vi "Convert_ERDs_Brass.vi"(0 "New Header?":bool, 7 "Array":T7[](array[typedef]) {"ERD Number" format="%.0x"}, 11 "Error In":errorcluster) -> (4 "All_ERD_Data_Bundled_Brass":T1, 15 "Error Out":errorcluster)   [LabVIEW 2016]
doc: "This VI parses the data from ERDs in correct format, units, etc. It handles all hex to dec conversions, hex to enum, and hex to boolean conversions.\n\nIf Raw Data from ERD is blank string, then it will output values from shift register."
uses:
  Common/LabVIEW GEA2 Toolkit/LabVIEW_GEA2_Toolkit.lvlibp/type defs/ERD Read Data Out.ctl
  type defs2/All_Bundled_Data_Brass.ctl
  Laundry Tool 1.0 Support/type defs/Version.ctl
  type defs2/ERD_Always_Show_Brass.ctl
  type defs2/CSV_File_String_Arrays.ctl
  type defs2/Fault Table Array.ctl
  Laundry Tool 1.0 Support/type defs/Fault_Table_Info.ctl
  Common/LabVIEW GEA2 Toolkit/LabVIEW_GEA2_Toolkit.lvlibp
panel:
  # "Software Version"
  # "UI"
  # "MC"
  # "INV"
  # "PERSONALITY"
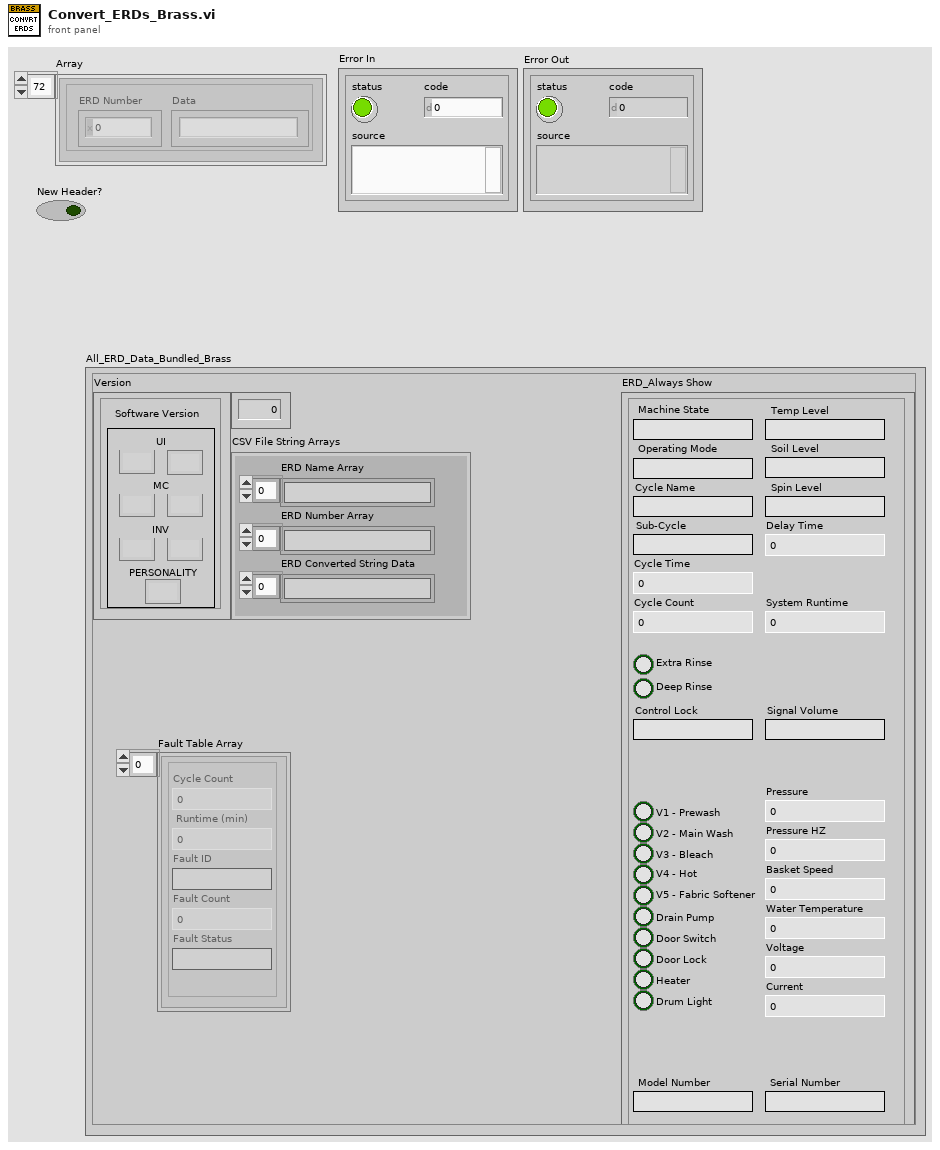
[diagram p1: front panel]
types:
  T1 = typedef "All_Bundled_Data_Brass.ctl" = cluster{"Version":T2, "ERD_Always Show":T3, "Personality Set":u8, "CSV File String Arrays":T4, "Fault Table Array ":T5}
  T2 = typedef "Version.ctl" = cluster{"UI Major":string, "UI Minor":string, "MC Minor":string, "MC Major":string, "Inverter Minor":string, "Inverter Major":string, "Personality":string}
  T3 = typedef "ERD_Always_Show_Brass.ctl" = cluster{"Machine State":string, "Cycle Count":u32, "Soil Level":string, "Spin Level":string, "Temp Level":string, "Delay Time":u16, "Sub-Cycle":string, "Cycle Name":string, "Model Number":string, "Serial Number":string, "System Runtime":u32, "Cycle Time":u16, "Operating Mode":string, "Deep Rinse":bool, "Extra Rinse":bool, "V1 - Prewash":bool, "V2 - Main Wash":bool, "V3 - Bleach":bool, "V4 - Hot":bool, "Drain Pump":bool, "Door Switch":bool, "Door Lock":bool, "Basket Speed":u16, "Water Temperature":dbl, "Voltage":u16, "Pressure":dbl, "Heater":bool, "Control Lock":string, "Signal Volume":string, "Current":u16, "Pressure HZ":dbl, "Drum Light":bool, "V5 - Fabric Softener":bool}
  T4 = typedef "CSV_File_String_Arrays.ctl" = cluster{"ERD Number Array":string[], "ERD Name Array":string[], "ERD Converted String Data":string[]}
  T5 = typedef "Fault Table Array.ctl" = T6[]
  T6 = typedef "Fault_Table_Info.ctl" = cluster{"Cycle Count":u32, " Runtime (min) ":u32, "Fault Status":string, "Fault ID":string, "Fault Count":u16}
  T7 = typedef "LabVIEW_GEA2_Toolkit.lvlibp/ERD Read Data Out.ctl" = cluster{"ERD Number":u16, "Data":string}
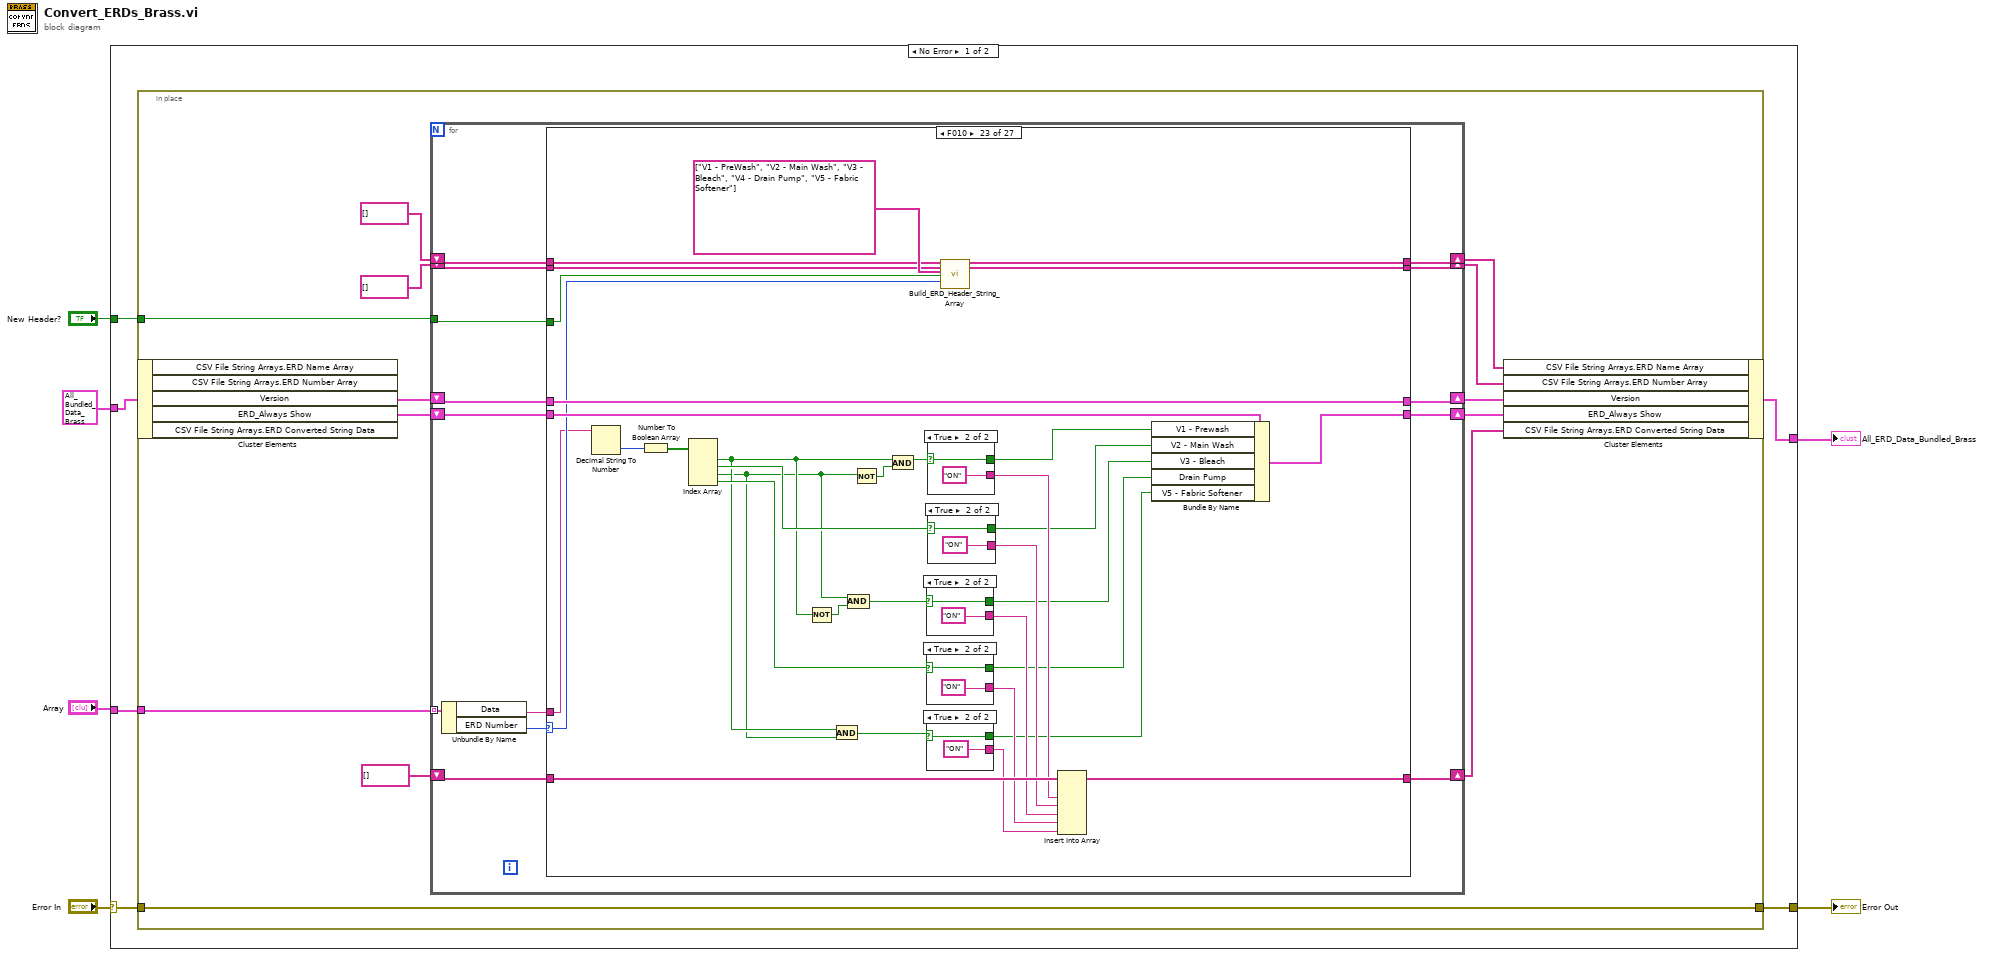
[diagram p0: block diagram]
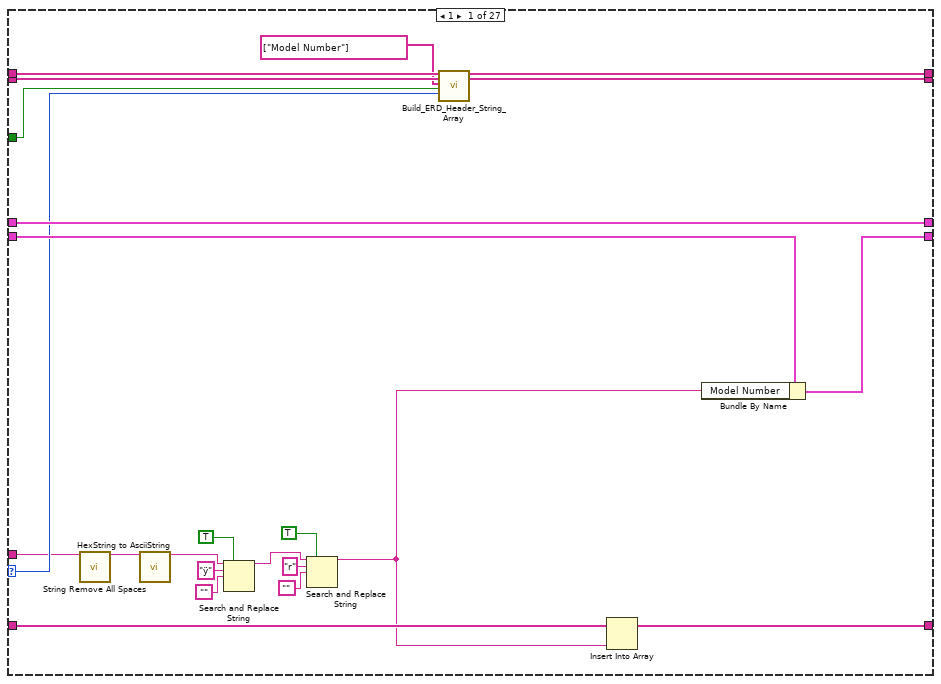
[diagram p2: hidden frame]
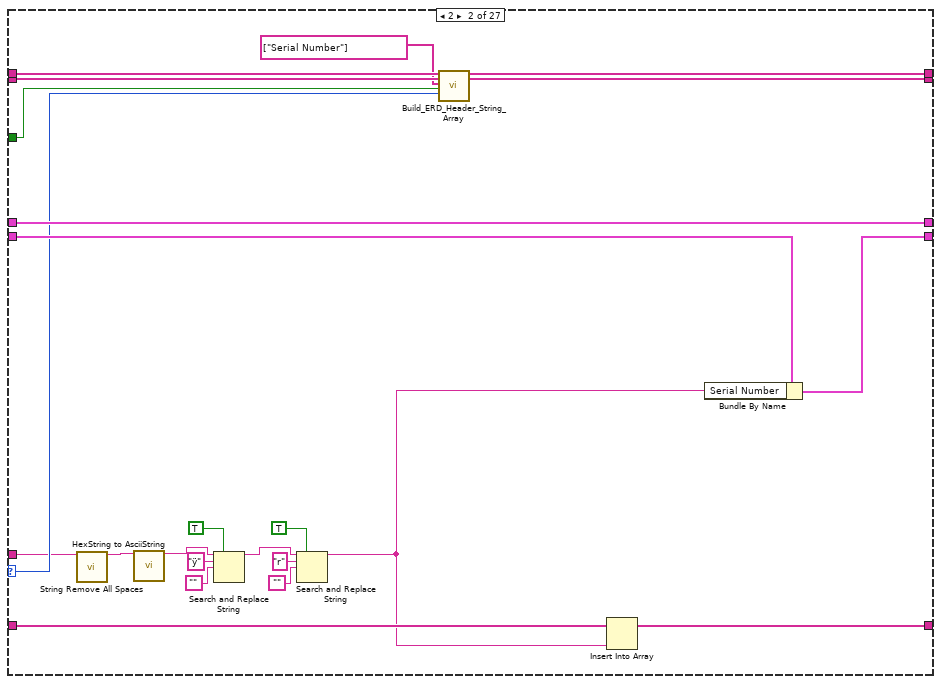
[diagram p3: hidden frame]
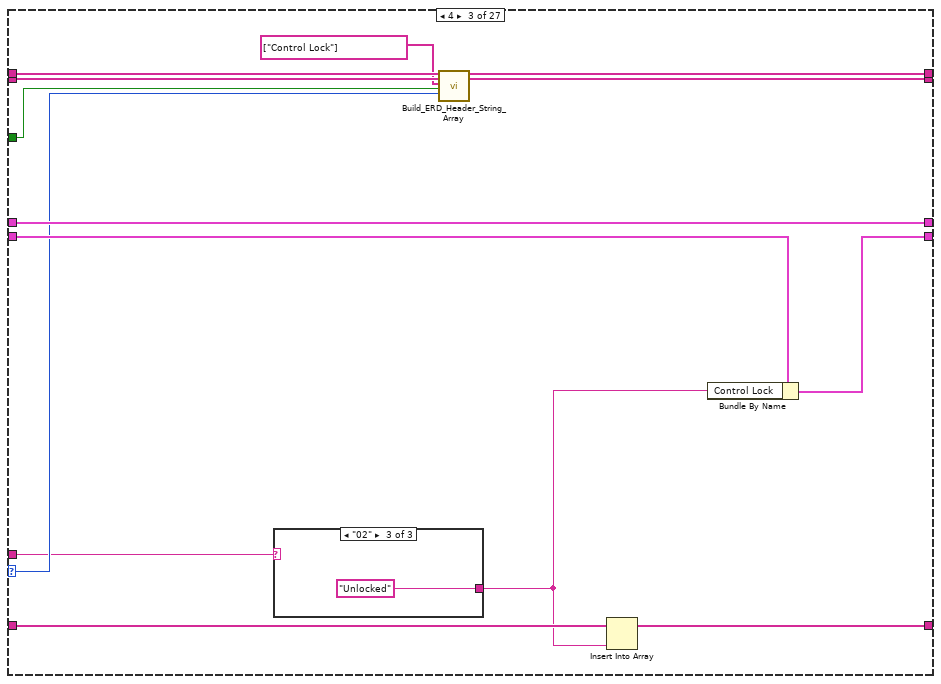
[diagram p4: hidden frame]
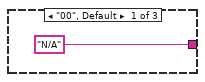
[diagram p5: hidden frame]
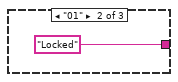
[diagram p6: hidden frame]
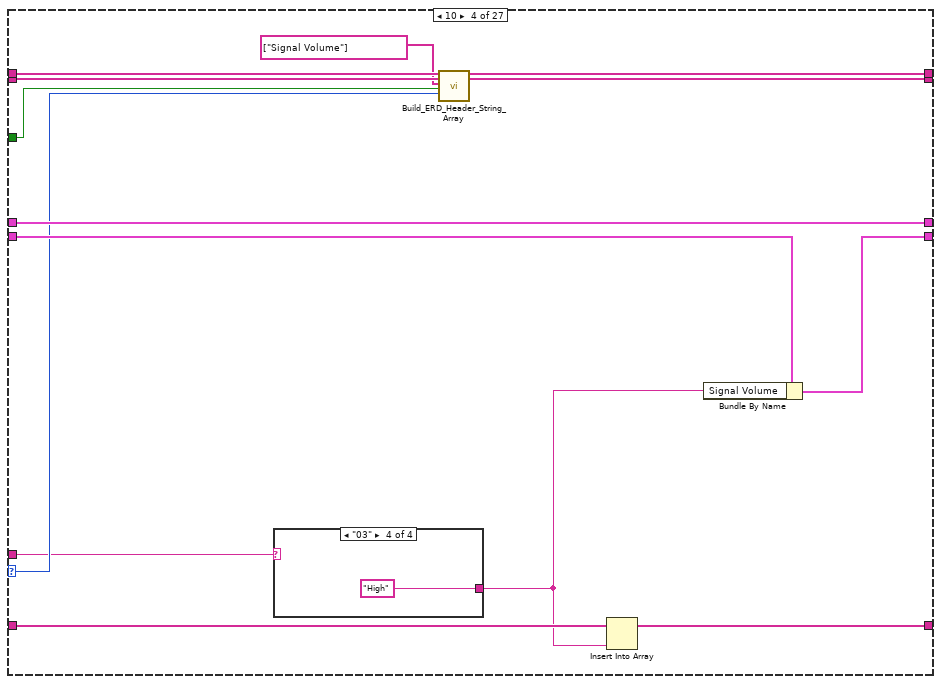
[diagram p7: hidden frame]
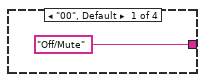
[diagram p8: hidden frame]
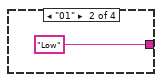
[diagram p9: hidden frame]
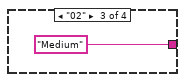
[diagram p10: hidden frame]
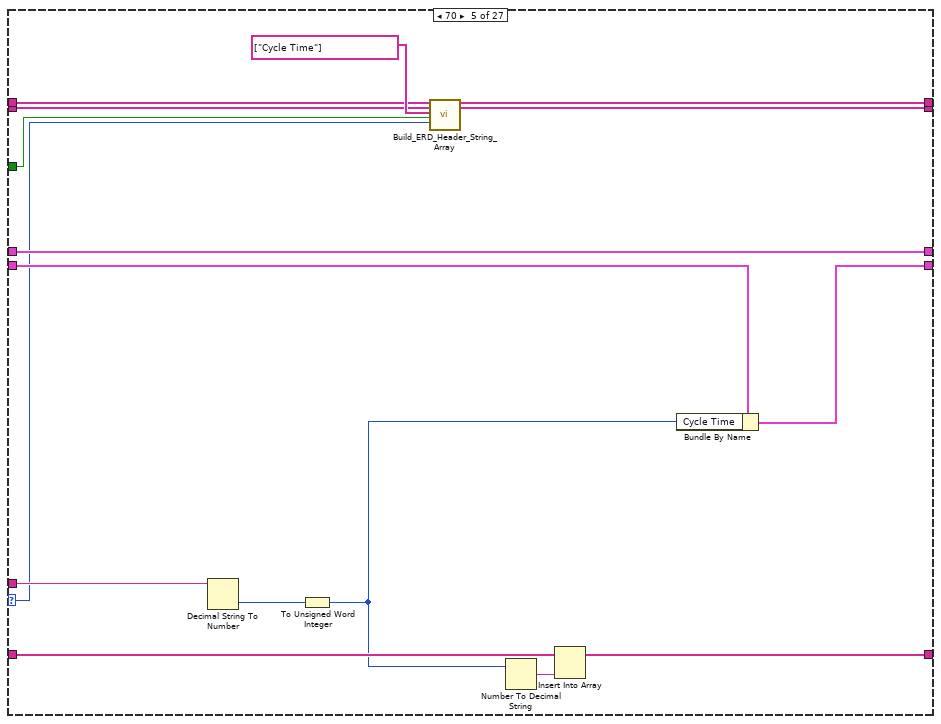
[diagram p11: hidden frame]
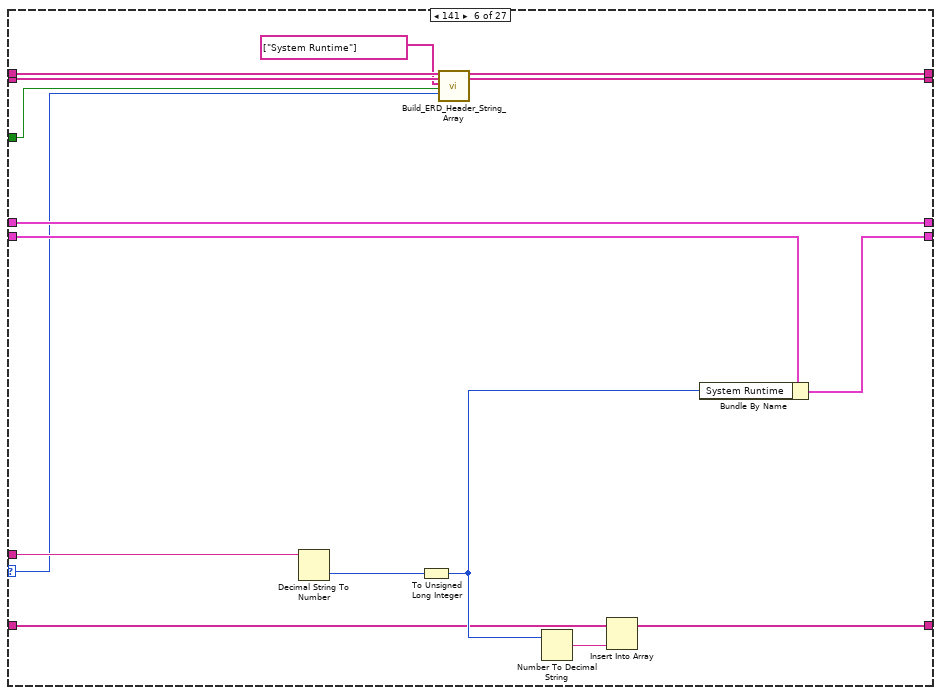
[diagram p12: hidden frame]
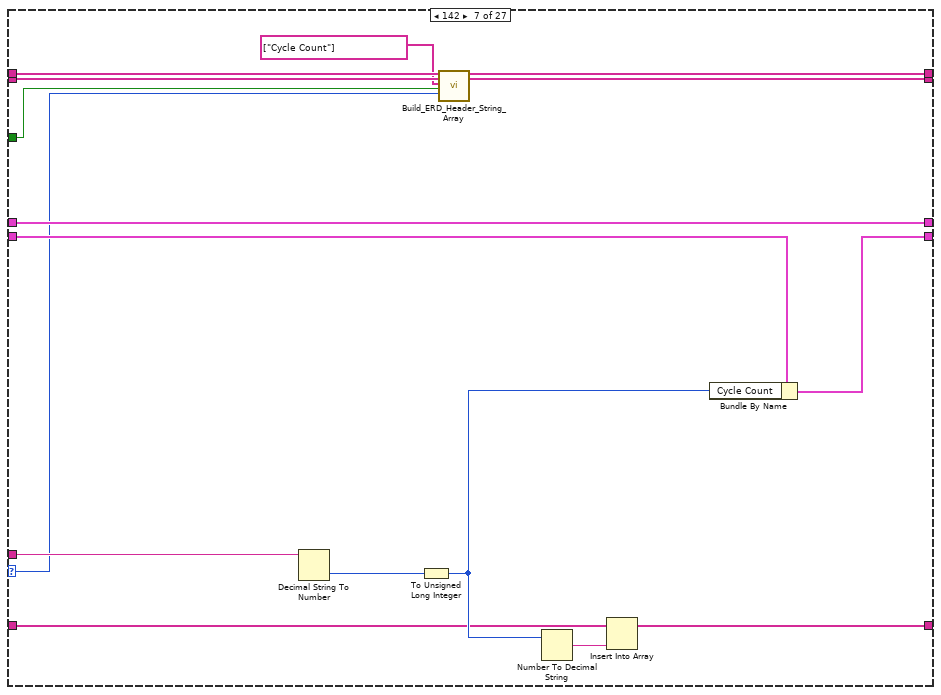
[diagram p13: hidden frame]
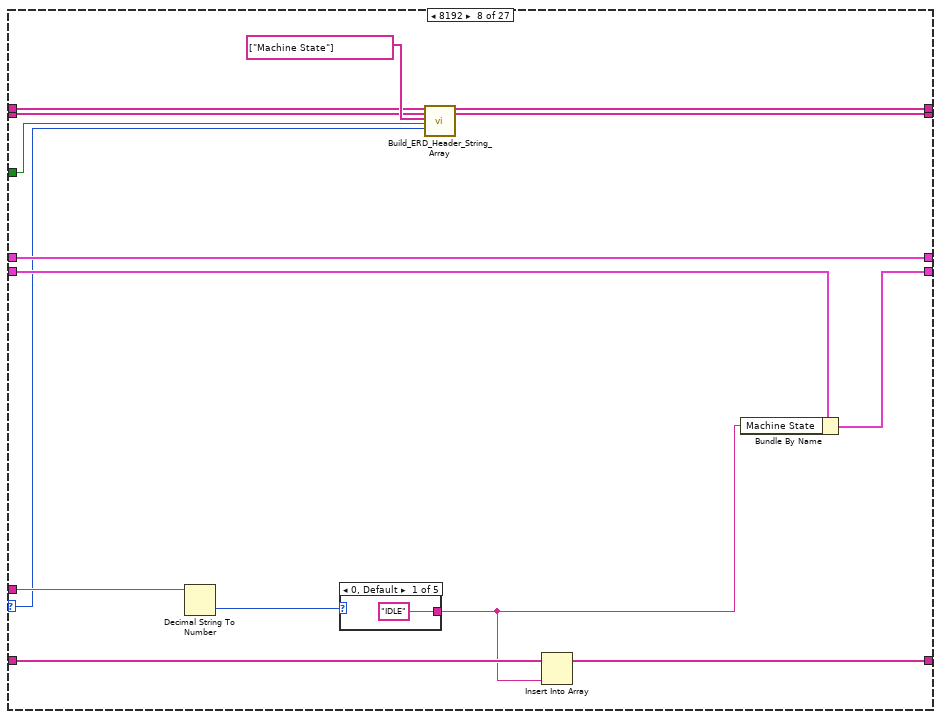
[diagram p14: hidden frame]
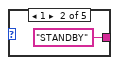
[diagram p15: hidden frame]
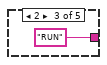
[diagram p16: hidden frame]
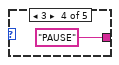
[diagram p17: hidden frame]
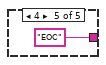
[diagram p18: hidden frame]
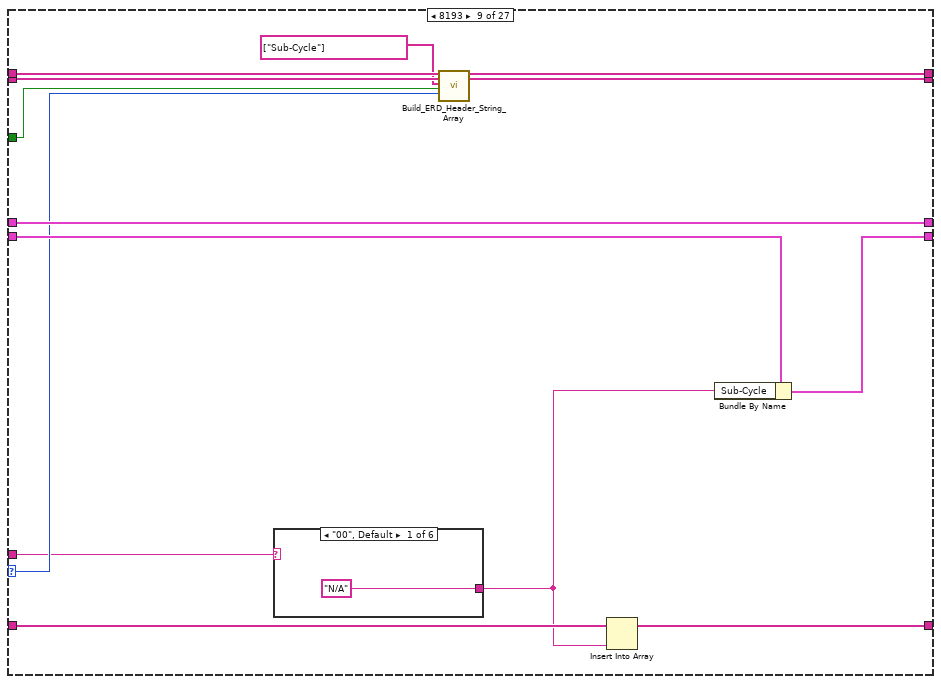
[diagram p19: hidden frame]
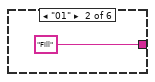
[diagram p20: hidden frame]
diagram:
  n1 = case shown="No Error" "Error In" {
    selector: "Error In" -> [w9 w657]
    tunnel: "Array" -> [w12 _]
    tunnel: [w10 w656] -> w4
    tunnel: T1 {"Version"={"UI Major"="", "UI Minor"="", "MC Minor"="", "MC Major"="", "Inverter Minor"="", "Inverter Major"="", "Personality"=""}, "ERD_Always Show"={"Machine State"="", "Cycle Count"=0, "Soil Level"="", "Spin Level"="", "Temp Level"="", "Delay Time"=0, "Sub-Cycle"="", "Cycle Name"="", "Model Number"="", "Serial Number"="", "System Runtime"=0, "Cycle Time"=0, "Operating Mode"="", "Deep Rinse"=FALSE, "Extra Rinse"=FALSE, "V1 - Prewash"=FALSE, "V2 - Main Wash"=FALSE, "V3 - Bleach"=FALSE, "V4 - Hot"=FALSE, "Drain Pump"=FALSE, "Door Switch"=FALSE, "Door Lock"=FALSE, "Basket Speed"=0, "Water Temperature"=0.0, "Voltage"=0, "Pressure"=0.0, "Heater"=FALSE, "Control Lock"="", "Signal Volume"="", "Current"=0, "Pressure HZ"=0.0, "Drum Light"=FALSE, "V5 - Fabric Softener"=FALSE}, "Personality Set"=0, "CSV File String Arrays"={"ERD Number Array"=[], "ERD Name Array"=[], "ERD Converted String Data"=[]}, "Fault Table Array "=[]} ("ERD_Data_Bundled_Out") -> [w11 w655]
    tunnel: [w8 w655] -> w3
    tunnel: "New Header?" -> [w7 _]
    frame No Error {
      n2 = in-place {
        in-place-border: w12 -> [w25]
        in-place-border: [w22] -> w10
        in-place-border: w9 -> [w22]
        in-place-border: w7 -> [w18]
        n3 = in-place-cluster #1(w11) -> ("Version"=w23:T2, "ERD_Always Show"=w24:T3)  [unwired: 3 out]
        n4 = for {
          tunnel: w25 -> [w39] mode=indexing
          shift-right: [w37] -> w20
          shift-left: w24 -> [w36]
          shift-right: [w34] -> w21
          shift-left: w23 -> [w35]
          shift-right: [w31] -> w13
          shift-left: string[] [] ("ERD String Data") -> [w32]
          tunnel: w18 -> [w30]
          shift-right: [w26] -> w14
          shift-left: string[] [] ("ERD String Data") -> [w29]
          shift-right: [w27] -> w15
          shift-left: string[] [] ("ERD String Data") -> [w28]
          n5 = Unbundle By Name(w39) -> ("Data"=w38:string, "ERD Number"=w33:u16)
          n6 = case shown="F010" w33 {
            selector: w33 -> [w53 w76 w90 w107 w121 w142 w158 w172 w193 w213 w270 w290 w311 w330 w344 w364 w387 w411 w442 w459 w478 w499 w537 w569 w588 w624 _]
            tunnel: w38 -> [w50 w73 w87 w104 w135 w152 w168 w180 w190 w210 w267 w304 w308 w327 w355 w375 w398 w421 w455 w472 w475 w498 w536 w583 w601 w603 _]
            tunnel: [w61 w84 w98 w115 w133 w150 w166 w183 w201 w221 w278 w302 w319 w338 w356 w376 w399 w422 w453 w470 w486 w509 w547 w581 w599 w635 w654] -> w37
            tunnel: w36 -> [w62 w85 w99 w116 w134 w151 w167 w182 w202 w222 w279 w303 w320 w339 w357 w377 w400 w423 w454 w471 w487 w510 w548 w582 w600 w635 w654]
            tunnel: w35 -> [w60 w83 w97 w114 w132 w149 w165 w179 w200 w220 w277 w301 w318 w337 w354 w374 w397 w420 w452 w469 w485 w508 w546 w580 w598 w637 w653]
            tunnel: [w60 w83 w97 w114 w132 w149 w165 w179 w200 w220 w277 w301 w318 w337 w354 w374 w397 w420 w452 w469 w485 w508 w546 w580 w598 w636 w653] -> w34
            tunnel: w32 -> [w58 w81 w95 w112 w125 w147 w163 w176 w198 w218 w275 w294 w316 w335 w348 w368 w391 w415 w446 w463 w483 w503 w541 w573 w592 w602 w651]
            tunnel: [w56 w79 w93 w110 w123 w145 w161 w174 w196 w216 w273 w292 w314 w333 w346 w366 w389 w413 w444 w461 w481 w501 w539 w571 w590 w626 w651] -> w31
            tunnel: w30 -> [w54 w77 w91 w108 w122 w143 w159 w173 w194 w214 w271 w291 w312 w331 w345 w365 w388 w412 w443 w460 w479 w500 w538 w570 w589 w625 _]
            tunnel: w29 -> [w59 w82 w96 w113 w126 w148 w164 w177 w199 w219 w276 w295 w317 w336 w349 w369 w392 w416 w447 w464 w484 w504 w542 w574 w593 w628 w652]
            tunnel: w28 -> [w52 w75 w89 w106 w130 w138 w154 w171 w192 w212 w269 w299 w310 w329 w353 w373 w396 w419 w450 w467 w477 w507 w545 w578 w596 w631 w650]
            tunnel: [w51 w74 w88 w105 w129 w137 w153 w170 w191 w211 w268 w298 w309 w328 w352 w372 w395 w418 w449 w466 w476 w506 w544 w577 w595 w630 w650] -> w27
            tunnel: [w57 w80 w94 w111 w124 w146 w162 w175 w197 w217 w274 w293 w315 w334 w347 w367 w390 w414 w445 w462 w482 w502 w540 w572 w591 w627 w652] -> w26
            frame 1 {
              n7 = call "String Remove All Spaces.vi"("Input String"=w50) -> ("Spaces Removed"=w49:string)  [unwired: 13 in, 1 out]
              n8 = call "HexString to AsciiString.vi"("Hex String"=w49) -> ("ASCII String"=w45:string)  [unwired: 13 in, 1 out]
              n9 = Search and Replace String(replace all?=TRUE ("replace all? (F)"), input string=w45, search string="ÿ", replace string="") -> (result string=w41:string)  [unwired: 4 in, 3 out]
              n10 = Search and Replace String(replace all?=TRUE ("replace all? (F)"), input string=w41, search string="r", replace string="") -> (result string=w44:string)  [unwired: 4 in, 3 out]
              n11 = call "Build_ERD_Header_String_Array.vi"("ERD Name Array In"=w59, "ERD Number Array In"=w58, "ERD Name List"=string[] ["Model Number"], "New Header?"=w54, "ERD Number"=w53) -> ("ERD Name Array Out"=w57:string[], "ERD Number Array Out"=w56:string[])  [unwired: 13 in]
              n12 = Insert Into Array(array=w52, new element=w44) -> (w51:string[])  [unwired: 1 in]
              n13 = Bundle By Name(cluster=w62, "Model Number"=w44) -> (w61:T3)
            }
            frame 2 {
              n14 = call "String Remove All Spaces.vi"("Input String"=w73) -> ("Spaces Removed"=w72:string)  [unwired: 13 in, 1 out]
              n15 = call "HexString to AsciiString.vi"("Hex String"=w72) -> ("ASCII String"=w69:string)  [unwired: 13 in, 1 out]
              n16 = Search and Replace String(replace all?=TRUE ("replace all? (F)"), input string=w69, search string="ÿ", replace string="") -> (result string=w64:string)  [unwired: 4 in, 3 out]
              n17 = Search and Replace String(replace all?=TRUE ("replace all? (F)"), input string=w64, search string="r", replace string="") -> (result string=w63:string)  [unwired: 4 in, 3 out]
              n18 = call "Build_ERD_Header_String_Array.vi"("ERD Name Array In"=w82, "ERD Number Array In"=w81, "ERD Name List"=string[] ["Serial Number"], "New Header?"=w77, "ERD Number"=w76) -> ("ERD Name Array Out"=w80:string[], "ERD Number Array Out"=w79:string[])  [unwired: 13 in]
              n19 = Insert Into Array(array=w75, new element=w63) -> (w74:string[])  [unwired: 1 in]
              n20 = Bundle By Name(cluster=w85, "Serial Number"=w63) -> (w84:T3)
            }
            frame 4 {
              n21 = case shown="\"02\"" w87 {
                tunnel: ["N/A" "Locked" "Unlocked"] -> w86
                frame "00", Default {
                }
                frame "01" {
                }
                frame "02" {
                }
              }
              n22 = call "Build_ERD_Header_String_Array.vi"("ERD Name Array In"=w96, "ERD Number Array In"=w95, "ERD Name List"=string[] ["Control Lock"], "New Header?"=w91, "ERD Number"=w90) -> ("ERD Name Array Out"=w94:string[], "ERD Number Array Out"=w93:string[])  [unwired: 13 in]
              n23 = Insert Into Array(array=w89, new element=w86) -> (w88:string[])  [unwired: 1 in]
              n24 = Bundle By Name(cluster=w99, "Control Lock"=w86) -> (w98:T3)
            }
            frame 10 {
              n25 = case shown="\"03\"" w104 {
                tunnel: ["Off/Mute" "Low" "Medium" "High"] -> w103
                frame "00", Default {
                }
                frame "01" {
                }
                frame "02" {
                }
                frame "03" {
                }
              }
              n26 = call "Build_ERD_Header_String_Array.vi"("ERD Name Array In"=w113, "ERD Number Array In"=w112, "ERD Name List"=string[] ["Signal Volume"], "New Header?"=w108, "ERD Number"=w107) -> ("ERD Name Array Out"=w111:string[], "ERD Number Array Out"=w110:string[])  [unwired: 13 in]
              n27 = Insert Into Array(array=w106, new element=w103) -> (w105:string[])  [unwired: 1 in]
              n28 = Bundle By Name(cluster=w116, "Signal Volume"=w103) -> (w115:T3)
            }
            frame 70 {
              n29 = Decimal String To Number(string=w135) -> (number=w136:i32)  [unwired: 2 in, 1 out]
              n30 = To Unsigned Word Integer(number=w136) -> (unsigned 16bit integer=w128:u16)
              n31 = call "Build_ERD_Header_String_Array.vi"("ERD Name Array In"=w126, "ERD Number Array In"=w125, "ERD Name List"=string[] ["Cycle Time"], "New Header?"=w122, "ERD Number"=w121) -> ("ERD Name Array Out"=w124:string[], "ERD Number Array Out"=w123:string[])  [unwired: 13 in]
              n32 = Number To Decimal String(number=w128) -> (decimal integer string=w131:string)  [unwired: 1 in]
              n33 = Insert Into Array(array=w130, new element=w131) -> (w129:string[])  [unwired: 1 in]
              n34 = Bundle By Name(cluster=w134, "Cycle Time"=w128) -> (w133:T3)
            }
            frame 141 {
              n35 = Decimal String To Number(string=w152) -> (number=w140:i32)  [unwired: 2 in, 1 out]
              n36 = To Unsigned Long Integer(number=w140) -> (unsigned 32bit integer=w139:u32)
              n37 = call "Build_ERD_Header_String_Array.vi"("ERD Name Array In"=w148, "ERD Number Array In"=w147, "ERD Name List"=string[] ["System Runtime"], "New Header?"=w143, "ERD Number"=w142) -> ("ERD Name Array Out"=w146:string[], "ERD Number Array Out"=w145:string[])  [unwired: 13 in]
              n38 = Number To Decimal String(number=w139) -> (decimal integer string=w141:string)  [unwired: 1 in]
              n39 = Insert Into Array(array=w138, new element=w141) -> (w137:string[])  [unwired: 1 in]
              n40 = Bundle By Name(cluster=w151, "System Runtime"=w139) -> (w150:T3)
            }
            frame 142 {
              n41 = Decimal String To Number(string=w168) -> (number=w156:i32)  [unwired: 2 in, 1 out]
              n42 = To Unsigned Long Integer(number=w156) -> (unsigned 32bit integer=w155:u32)
              n43 = call "Build_ERD_Header_String_Array.vi"("ERD Name Array In"=w164, "ERD Number Array In"=w163, "ERD Name List"=string[] ["Cycle Count"], "New Header?"=w159, "ERD Number"=w158) -> ("ERD Name Array Out"=w162:string[], "ERD Number Array Out"=w161:string[])  [unwired: 13 in]
              n44 = Number To Decimal String(number=w155) -> (decimal integer string=w157:string)  [unwired: 1 in]
              n45 = Insert Into Array(array=w154, new element=w157) -> (w153:string[])  [unwired: 1 in]
              n46 = Bundle By Name(cluster=w167, "Cycle Count"=w155) -> (w166:T3)
            }
            frame 8192 {
              n47 = Decimal String To Number(string=w180) -> (number=w181:i32)  [unwired: 2 in, 1 out]
              n48 = case shown="0, Default" w181 {
                tunnel: ["IDLE" "STANDBY" "RUN" "PAUSE" "EOC"] -> w169
                frame 0, Default {
                }
                frame 1 {
                }
                frame 2 {
                }
                frame 3 {
                }
                frame 4 {
                }
              }
              n49 = call "Build_ERD_Header_String_Array.vi"("ERD Name Array In"=w177, "ERD Number Array In"=w176, "ERD Name List"=string[] ["Machine State"], "New Header?"=w173, "ERD Number"=w172) -> ("ERD Name Array Out"=w175:string[], "ERD Number Array Out"=w174:string[])  [unwired: 13 in]
              n50 = Insert Into Array(array=w171, new element=w169) -> (w170:string[])  [unwired: 1 in]
              n51 = Bundle By Name(cluster=w182, "Machine State"=w169) -> (w183:T3)
            }
            frame 8193 {
              n52 = case shown="\"00\", Default" w190 {
                tunnel: ["N/A" "Fill" "Soak" "Wash" "Rinse" "Spin"] -> w189
                frame "00", Default {
                }
                frame "01" {
                }
                frame "02" {
                }
                frame "03" {
                }
                frame "04" {
                }
                frame "05" {
                }
              }
              n53 = call "Build_ERD_Header_String_Array.vi"("ERD Name Array In"=w199, "ERD Number Array In"=w198, "ERD Name List"=string[] ["Sub-Cycle"], "New Header?"=w194, "ERD Number"=w193) -> ("ERD Name Array Out"=w197:string[], "ERD Number Array Out"=w196:string[])  [unwired: 13 in]
              n54 = Insert Into Array(array=w192, new element=w189) -> (w191:string[])  [unwired: 1 in]
              n55 = Bundle By Name(cluster=w202, "Sub-Cycle"=w189) -> (w201:T3)
            }
            frame 8202 {
              n56 = case shown="\"19\"" w210 {
                tunnel: ["Not Defined" "Basket Clean" "Drain & Spin" "Quick Rinse" "Bulky Items" "Sanitize" "Towels & Sheets" "Steam Refresh" "Normal/Mixed" "Whites" "Dark Colors" "Jeans" "Hand Wash" "Delicates" "Speed Wash" "Heavy Duty" "Allergen" "Power Clean" "Rinse & Spin" "Single Item" "Colors" "Cold Wash" "Water on Demand" "Tub Clean" "Casuals w/ Steam" "Stain Wash w/ Steam" "Cottons" "Easy Care" "Active Wear" "Timed Dry" "Dewrinkle" "Air Fluff" "Steam Refresh" "Steam Dewrinkle" "Speed Dry" "Mixed" "Quick Dry" "Casuals" "Warm Up" "Energy Saver" "Antibacterial" "Rack Dry" "Baby Care"] -> w209
                frame "00", Default {
                }
                frame "01" {
                }
                frame "02" {
                }
                frame "03" {
                }
                frame "04" {
                }
                frame "05" {
                }
                frame "06" {
                }
                frame "07" {
                }
                frame "08" {
                }
                frame "09" {
                }
                frame "0A" {
                }
                frame "0B" {
                }
                frame "0C" {
                }
                frame "0D" {
                }
                frame "0E" {
                }
                frame "0F" {
                }
                frame "10" {
                }
                frame "11" {
                }
                frame "12" {
                }
                frame "13" {
                }
                frame "14" {
                }
                frame "15" {
                }
                frame "16" {
                }
                frame "17" {
                }
                frame "18" {
                }
                frame "19" {
                }
                frame "80" {
                }
                frame "81" {
                }
                frame "82" {
                }
                frame "83" {
                }
                frame "84" {
                }
                frame "85" {
                }
                frame "86" {
                }
                frame "87" {
                }
                frame "88" {
                }
                frame "89" {
                }
                frame "8A" {
                }
                frame "8B" {
                }
                frame "8C" {
                }
                frame "8D" {
                }
                frame "8E" {
                }
                frame "8F" {
                }
                frame "90" {
                }
              }
              n57 = call "Build_ERD_Header_String_Array.vi"("ERD Name Array In"=w219, "ERD Number Array In"=w218, "ERD Name List"=string[] ["Cycle Name"], "New Header?"=w214, "ERD Number"=w213) -> ("ERD Name Array Out"=w217:string[], "ERD Number Array Out"=w216:string[])  [unwired: 13 in]
              n58 = Insert Into Array(array=w212, new element=w209) -> (w211:string[])  [unwired: 1 in]
              n59 = Bundle By Name(cluster=w222, "Cycle Name"=w209) -> (w221:T3)
            }
            frame 8206 {
              n60 = case shown="\"09\"" w267 {
                tunnel: ["Consumer Mode" "Service Mode" "factory/EOL Mode" "Continuous Cycle Mode" "Rapid Relay Mode" "FCT Mode" "Model Plug" "Demo Mode" "Consumer Error Mode" "Floor Type Selection Mode"] -> w266
                frame "00", Default {
                }
                frame "01" {
                }
                frame "02" {
                }
                frame "03" {
                }
                frame "04" {
                }
                frame "05" {
                }
                frame "06" {
                }
                frame "07" {
                }
                frame "08" {
                }
                frame "09" {
                }
              }
              n61 = call "Build_ERD_Header_String_Array.vi"("ERD Name Array In"=w276, "ERD Number Array In"=w275, "ERD Name List"=string[] ["Operating Mode"], "New Header?"=w271, "ERD Number"=w270) -> ("ERD Name Array Out"=w274:string[], "ERD Number Array Out"=w273:string[])  [unwired: 13 in]
              n62 = Insert Into Array(array=w269, new element=w266) -> (w268:string[])  [unwired: 1 in]
              n63 = Bundle By Name(cluster=w279, "Operating Mode"=w266) -> (w278:T3)
            }
            frame 8208 {
              n64 = Decimal String To Number(string=w304) -> (number=w305:i32)  [unwired: 2 in, 1 out]
              n65 = To Unsigned Word Integer(number=w305) -> (unsigned 16bit integer=w297:u16)
              n66 = call "Build_ERD_Header_String_Array.vi"("ERD Name Array In"=w295, "ERD Number Array In"=w294, "ERD Name List"=string[] ["Delay Time"], "New Header?"=w291, "ERD Number"=w290) -> ("ERD Name Array Out"=w293:string[], "ERD Number Array Out"=w292:string[])  [unwired: 13 in]
              n67 = Number To Decimal String(number=w297) -> (decimal integer string=w300:string)  [unwired: 1 in]
              n68 = Insert Into Array(array=w299, new element=w300) -> (w298:string[])  [unwired: 1 in]
              n69 = Bundle By Name(cluster=w303, "Delay Time"=w297) -> (w302:T3)
            }
            frame 8210 {
              n70 = case shown="\"00\", Default" w308 {
                tunnel: ["Open" "Closed"] -> w307
                tunnel: [FALSE TRUE] -> w306
                frame "00", Default {
                }
                frame "01" {
                }
              }
              n71 = call "Build_ERD_Header_String_Array.vi"("ERD Name Array In"=w317, "ERD Number Array In"=w316, "ERD Name List"=string[] ["Door Switch"], "New Header?"=w312, "ERD Number"=w311) -> ("ERD Name Array Out"=w315:string[], "ERD Number Array Out"=w314:string[])  [unwired: 13 in]
              n72 = Insert Into Array(array=w310, new element=w307) -> (w309:string[])  [unwired: 1 in]
              n73 = Bundle By Name(cluster=w320, "Door Switch"=w306) -> (w319:T3)
            }
            frame 8211 {
              n74 = case shown="\"01\"" w327 {
                tunnel: ["Unlocked" "Locked"] -> w326
                tunnel: [FALSE TRUE] -> w325
                frame "00", Default {
                }
                frame "01" {
                }
              }
              n75 = call "Build_ERD_Header_String_Array.vi"("ERD Name Array In"=w336, "ERD Number Array In"=w335, "ERD Name List"=string[] ["Door Lock"], "New Header?"=w331, "ERD Number"=w330) -> ("ERD Name Array Out"=w334:string[], "ERD Number Array Out"=w333:string[])  [unwired: 13 in]
              n76 = Insert Into Array(array=w329, new element=w326) -> (w328:string[])  [unwired: 1 in]
              n77 = Bundle By Name(cluster=w339, "Door Lock"=w325) -> (w338:T3)
            }
            frame 8213 {
              n78 = case shown="\"00\"" w355 {
                selector: w355 -> [w358 _ _ _ _ _]
                tunnel: [w358 "Extra Light" "Light" "Normal" "Heavy" "Extra Heavy"] -> w351
                frame Default {
                }
                frame "00" {
                }
                frame "01" {
                }
                frame "02" {
                }
                frame "03" {
                }
                frame "04" {
                }
              }
              n79 = call "Build_ERD_Header_String_Array.vi"("ERD Name Array In"=w349, "ERD Number Array In"=w348, "ERD Name List"=string[] ["Soil Level"], "New Header?"=w345, "ERD Number"=w344) -> ("ERD Name Array Out"=w347:string[], "ERD Number Array Out"=w346:string[])  [unwired: 13 in]
              n80 = Insert Into Array(array=w353, new element=w351) -> (w352:string[])  [unwired: 1 in]
              n81 = Bundle By Name(cluster=w357, "Soil Level"=w351) -> (w356:T3)
            }
            frame 8214 {
              n82 = case shown="\"22\"" w375 {
                selector: w375 -> [w378 _ _ _ _ _ _ _ _]
                tunnel: [w378 "Disabled" "Tap Cold" "Cold" "Cool" "Colors" "Warm" "Hot" "Extra Hot"] -> w371
                frame Default {
                }
                frame "06" {
                }
                frame "16" {
                }
                frame "17" {
                }
                frame "18" {
                }
                frame "19" {
                }
                frame "20" {
                }
                frame "21" {
                }
                frame "22" {
                }
              }
              n83 = call "Build_ERD_Header_String_Array.vi"("ERD Name Array In"=w369, "ERD Number Array In"=w368, "ERD Name List"=string[] ["Temp Level"], "New Header?"=w365, "ERD Number"=w364) -> ("ERD Name Array Out"=w367:string[], "ERD Number Array Out"=w366:string[])  [unwired: 13 in]
              n84 = Insert Into Array(array=w373, new element=w371) -> (w372:string[])  [unwired: 1 in]
              n85 = Bundle By Name(cluster=w377, "Temp Level"=w371) -> (w376:T3)
            }
            frame 8215 {
              n86 = case shown="\"5\"" w398 {
                selector: w398 -> [w401 _ _ _ _ _ _]
                tunnel: [w401 "No Spin" "Low" "Medium" "High" "Extra High" "Disable"] -> w394
                frame Default {
                }
                frame "0" {
                }
                frame "1" {
                }
                frame "2" {
                }
                frame "3" {
                }
                frame "4" {
                }
                frame "5" {
                }
              }
              n87 = call "Build_ERD_Header_String_Array.vi"("ERD Name Array In"=w392, "ERD Number Array In"=w391, "ERD Name List"=string[] ["Spin Level"], "New Header?"=w388, "ERD Number"=w387) -> ("ERD Name Array Out"=w390:string[], "ERD Number Array Out"=w389:string[])  [unwired: 13 in]
              n88 = Insert Into Array(array=w396, new element=w394) -> (w395:string[])  [unwired: 1 in]
              n89 = Bundle By Name(cluster=w400, "Spin Level"=w394) -> (w399:T3)
            }
            frame 8216 {
              n90 = case shown="\"3\"" w421 {
                selector: w421 -> [w424 _ _ _ _]
                tunnel: [w424 "0 - Deep Rinse OFF - Extra Rinse OFF" "1 - Deep Rinse ON - Extra Rinse OFF" "2 - Deep Rinse OFF - Extra Rinse ON" "3 - Deep Rinse ON - Extra Rinse ON"] -> w410
                tunnel: [FALSE FALSE TRUE FALSE TRUE] -> w409
                tunnel: [FALSE FALSE FALSE TRUE TRUE] -> w408
                frame Default {
                }
                frame "0" {
                }
                frame "1" {
                }
                frame "2" {
                }
                frame "3" {
                }
              }
              n91 = call "Build_ERD_Header_String_Array.vi"("ERD Name Array In"=w416, "ERD Number Array In"=w415, "ERD Name List"=string[] ["Rinse Options"], "New Header?"=w412, "ERD Number"=w411) -> ("ERD Name Array Out"=w414:string[], "ERD Number Array Out"=w413:string[])  [unwired: 13 in]
              n92 = Insert Into Array(array=w419, new element=w410) -> (w418:string[])  [unwired: 1 in]
              n93 = Bundle By Name(cluster=w423, "Deep Rinse"=w409, "Extra Rinse"=w408) -> (w422:T3)
            }
            frame 8258 {
              n94 = Decimal String To Number(string=w455) -> (number=w441:i32)  [unwired: 2 in, 1 out]
              n95 = Divide(x=w441, y=1000) -> (x/y=w439:dbl)
              n96 = call "Build_ERD_Header_String_Array.vi"("ERD Name Array In"=w447, "ERD Number Array In"=w446, "ERD Name List"=string[] ["Pressure"], "New Header?"=w443, "ERD Number"=w442) -> ("ERD Name Array Out"=w445:string[], "ERD Number Array Out"=w444:string[])  [unwired: 13 in]
              n97 = Number To Fractional String(number=w439) -> (F-format string=w451:string)  [unwired: 3 in]
              n98 = Insert Into Array(array=w450, new element=w451) -> (w449:string[])  [unwired: 1 in]
              n99 = Bundle By Name(cluster=w454, "Pressure"=w439) -> (w453:T3)
            }
            frame 8259 {
              n100 = Decimal String To Number(string=w472) -> (number=w458:i32)  [unwired: 2 in, 1 out]
              n101 = Divide(x=w458, y=10) -> (x/y=w456:dbl)
              n102 = call "Build_ERD_Header_String_Array.vi"("ERD Name Array In"=w464, "ERD Number Array In"=w463, "ERD Name List"=string[] ["Water Temperature"], "New Header?"=w460, "ERD Number"=w459) -> ("ERD Name Array Out"=w462:string[], "ERD Number Array Out"=w461:string[])  [unwired: 13 in]
              n103 = Number To Fractional String(number=w456) -> (F-format string=w468:string)  [unwired: 3 in]
              n104 = Insert Into Array(array=w467, new element=w468) -> (w466:string[])  [unwired: 1 in]
              n105 = Bundle By Name(cluster=w471, "Water Temperature"=w456) -> (w470:T3)
            }
            frame 61452 {
              n106 = case shown="\"01\"" w475 {
                tunnel: ["OFF" "ON"] -> w474
                tunnel: [FALSE TRUE] -> w473
                frame "00", Default {
                }
                frame "01" {
                }
              }
              n107 = call "Build_ERD_Header_String_Array.vi"("ERD Name Array In"=w484, "ERD Number Array In"=w483, "ERD Name List"=string[] ["Drum Light"], "New Header?"=w479, "ERD Number"=w478) -> ("ERD Name Array Out"=w482:string[], "ERD Number Array Out"=w481:string[])  [unwired: 13 in]
              n108 = Insert Into Array(array=w477, new element=w474) -> (w476:string[])  [unwired: 1 in]
              n109 = Bundle By Name(cluster=w487, "Drum Light"=w473) -> (w486:T3)
            }
            frame 61455 {
              n110 = Decimal String To Number(string=w498) -> (number=w497:i32)  [unwired: 2 in, 1 out]
              n111 = Number To Boolean Array(number=w497) -> (Boolean array=w496:bool[])
              n112 = Index Array(array=w496) -> (element #2=w493:bool, element #6=w492:bool)  [unwired: 6 in, 4 out]
              n113 = case shown="True" w493 {
                tunnel: ["OFF" "ON"] -> w495
                frame False {
                }
                frame True {
                }
              }
              n114 = case shown="True" w492 {
                tunnel: ["OFF" "ON"] -> w494
                frame False {
                }
                frame True {
                }
              }
              n115 = call "Build_ERD_Header_String_Array.vi"("ERD Name Array In"=w504, "ERD Number Array In"=w503, "ERD Name List"=string[] ["Heater", "V4 - Hot"], "New Header?"=w500, "ERD Number"=w499) -> ("ERD Name Array Out"=w502:string[], "ERD Number Array Out"=w501:string[])  [unwired: 13 in]
              n116 = Insert Into Array(array=w507, new element #1=w495, new element #2=w494) -> (w506:string[])  [unwired: 1 in]
              n117 = Bundle By Name(cluster=w510, "Heater"=w493, "V4 - Hot"=w492) -> (w509:T3)
            }
            frame 61456 {
              n118 = Decimal String To Number(string=w536) -> (number=w535:i32)  [unwired: 2 in, 1 out]
              n119 = Number To Boolean Array(number=w535) -> (Boolean array=w534:bool[])
              n120 = Index Array(array=w534) -> (element #1=w520:bool, element #2=w529:bool, element #3=w519:bool, element #4=w525:bool)  [unwired: 4 in]
              n121 = Not(x=w520) -> (.not. x?=w524:bool)
              n122 = And(x=w520, y=w519) -> (x .and. y?=w521:bool)
              n123 = And(x=w519, y=w524) -> (x .and. y?=w523:bool)
              n124 = Not(x=w519) -> (.not. x?=w527:bool)
              n125 = And(x=w520, y=w527) -> (x .and. y?=w528:bool)
              n126 = case shown="True" w523 {
                selector: w523 -> [w557 w559]
                tunnel: ["OFF" "ON"] -> w531
                tunnel: [w557 w559] -> w522
                frame False {
                }
                frame True {
                }
              }
              n127 = case shown="True" w525 {
                selector: w525 -> [w553 w555]
                tunnel: ["OFF" "ON"] -> w530
                tunnel: [w553 w555] -> w517
                frame False {
                }
                frame True {
                }
              }
              n128 = case shown="True" w521 {
                selector: w521 -> [w549 w551]
                tunnel: ["OFF" "ON"] -> w515
                tunnel: [w549 w551] -> w518
                frame False {
                }
                frame True {
                }
              }
              n129 = case shown="True" w528 {
                selector: w528 -> [w565 w567]
                tunnel: ["OFF" "ON"] -> w533
                tunnel: [w565 w567] -> w526
                frame False {
                }
                frame True {
                }
              }
              n130 = case shown="True" w529 {
                selector: w529 -> [w561 w563]
                tunnel: ["OFF" "ON"] -> w532
                tunnel: [w561 w563] -> w516
                frame False {
                }
                frame True {
                }
              }
              n131 = call "Build_ERD_Header_String_Array.vi"("ERD Name Array In"=w542, "ERD Number Array In"=w541, "ERD Name List"=string[] ["V1 - PreWash", "V2 - Main Wash", "V3 - Bleach", "V4 - Drain Pump", "V5 - Fabric Softener"], "New Header?"=w538, "ERD Number"=w537) -> ("ERD Name Array Out"=w540:string[], "ERD Number Array Out"=w539:string[])  [unwired: 13 in]
              n132 = Insert Into Array(array=w545, new element #1=w533, new element #2=w532, new element #3=w531, new element #4=w530, new element #5=w515) -> (w544:string[])  [unwired: 1 in]
              n133 = Bundle By Name(cluster=w548, "V1 - Prewash"=w526, "V2 - Main Wash"=w516, "V3 - Bleach"=w522, "Drain Pump"=w517, "V5 - Fabric Softener"=w518) -> (w547:T3)
            }
            frame 61457 {
              n134 = Decimal String To Number(string=w583) -> (number=w584:i32)  [unwired: 2 in, 1 out]
              n135 = To Unsigned Word Integer(number=w584) -> (unsigned 16bit integer=w576:u16)
              n136 = call "Build_ERD_Header_String_Array.vi"("ERD Name Array In"=w574, "ERD Number Array In"=w573, "ERD Name List"=string[] ["Basket Speed"], "New Header?"=w570, "ERD Number"=w569) -> ("ERD Name Array Out"=w572:string[], "ERD Number Array Out"=w571:string[])  [unwired: 13 in]
              n137 = Number To Decimal String(number=w576) -> (decimal integer string=w579:string)  [unwired: 1 in]
              n138 = Insert Into Array(array=w578, new element=w579) -> (w577:string[])  [unwired: 1 in]
              n139 = Bundle By Name(cluster=w582, "Basket Speed"=w576) -> (w581:T3)
            }
            frame 61458 {
              n140 = Decimal String To Number(string=w601) -> (number=w587:i32)  [unwired: 2 in, 1 out]
              n141 = Divide(x=w587, y=100) -> (x/y=w585:dbl)
              n142 = call "Build_ERD_Header_String_Array.vi"("ERD Name Array In"=w593, "ERD Number Array In"=w592, "ERD Name List"=string[] ["Pressure Hz"], "New Header?"=w589, "ERD Number"=w588) -> ("ERD Name Array Out"=w591:string[], "ERD Number Array Out"=w590:string[])  [unwired: 13 in]
              n143 = Number To Fractional String(number=w585) -> (F-format string=w597:string)  [unwired: 3 in]
              n144 = Insert Into Array(array=w596, new element=w597) -> (w595:string[])  [unwired: 1 in]
              n145 = Bundle By Name(cluster=w600, "Pressure HZ"=w585) -> (w599:T3)
            }
            frame 61460 {
              w613 = 2 ("length (rest)")
              n146 = String Subset(string=w603, offset (0)=0 ("length (rest)"), length (rest)=w613) -> (substring=w649:string)
              n147 = String Subset(string=w603, offset (0)=3 ("length (rest)"), length (rest)=w613) -> (substring=w645:string)
              n148 = String Subset(string=w603, offset (0)=6 ("length (rest)"), length (rest)=w613) -> (substring=w640:string)
              n149 = String Subset(string=w603, offset (0)=9 ("length (rest)"), length (rest)=w613) -> (substring=w639:string)
              n150 = String Subset(string=w603, offset (0)=12 ("length (rest)"), length (rest)=w613) -> (substring=w622:string)
              n151 = String Subset(string=w603, offset (0)=15 ("length (rest)"), length (rest)=w613) -> (substring=w617:string)
              n152 = String Subset(string=w603, offset (0)=18 ("length (rest)"), length (rest)=w613) -> (substring=w616:string)
              n153 = Hexadecimal String To Number(string=w649) -> (number=w644:u32)  [unwired: 2 in, 1 out]
              n154 = Hexadecimal String To Number(string=w645) -> (number=w643:u32)  [unwired: 2 in, 1 out]
              n155 = Hexadecimal String To Number(string=w640) -> (number=w642:u32)  [unwired: 2 in, 1 out]
              n156 = Hexadecimal String To Number(string=w639) -> (number=w641:u32)  [unwired: 2 in, 1 out]
              n157 = Hexadecimal String To Number(string=w622) -> (number=w621:u32)  [unwired: 2 in, 1 out]
              n158 = Hexadecimal String To Number(string=w617) -> (number=w618:u32)  [unwired: 2 in, 1 out]
              n159 = Hexadecimal String To Number(string=w616) -> (number=w615:u32)  [unwired: 2 in, 1 out]
              n160 = Number To Decimal String(number=w644) -> (decimal integer string=w633:string)  [unwired: 1 in]
              n161 = Number To Decimal String(number=w643) -> (decimal integer string=w632:string)  [unwired: 1 in]
              n162 = Number To Decimal String(number=w642) -> (decimal integer string=w610:string)  [unwired: 1 in]
              n163 = Number To Decimal String(number=w641) -> (decimal integer string=w609:string)  [unwired: 1 in]
              n164 = Number To Decimal String(number=w621) -> (decimal integer string=w608:string)  [unwired: 1 in]
              n165 = Number To Decimal String(number=w618) -> (decimal integer string=w607:string)  [unwired: 1 in]
              n166 = Number To Decimal String(number=w615) -> (decimal integer string=w604:string)  [unwired: 1 in]
              n167 = call "Build_ERD_Header_String_Array.vi"("ERD Name Array In"=w628, "ERD Number Array In"=w602, "ERD Name List"=string[] ["UI Verion", "MC Version", "Inv Version", "Personality"], "New Header?"=w625, "ERD Number"=w624) -> ("ERD Name Array Out"=w627:string[], "ERD Number Array Out"=w626:string[])  [unwired: 13 in]
              n168 = Concatenate Strings(w608, "." ("element"), w607) -> (w605:string)
              n169 = Concatenate Strings(w610, "." ("element"), w609) -> (w606:string)
              n170 = Concatenate Strings(w633, "." ("element"), w632) -> (w623:string)
              n171 = Bundle By Name(cluster=w637, "UI Major"=w633, "UI Minor"=w632, "MC Major"=w610, "MC Minor"=w609, "Inverter Major"=w608, "Inverter Minor"=w607, "Personality"=w604) -> (w636:T2)
              n172 = Insert Into Array(array=w631, new element #1=w623, new element #2=w606, new element #3=w605, new element #4=w604) -> (w630:string[])  [unwired: 1 in]
            }
            frame Default {
            }
          }
        }
        n173 = in-place-cluster #1("CSV File String Arrays.ERD Name Array"=w14, "CSV File String Arrays.ERD Number Array"=w13, "Version"=w21, "ERD_Always Show"=w20, "CSV File String Arrays.ERD Converted String Data"=w15) -> (w8:T1)
      }
    }
    frame Error {
      n174 = Unbundle By Name(w657) -> ("code"=w661:i32, "status"=w662:bool, "source"=w659:string)
      n175 = Equal?(x=w661, y=-5006) -> (x = y?=w665:bool)
      n176 = case shown="True" w665 {
        tunnel: [w669 FALSE] -> w663
        tunnel: w662 -> [w669 _]
        tunnel: w661 -> [w668 w671]
        tunnel: [w668 w671] -> w660
        tunnel: [w667 w670] -> w658
        tunnel: w659 -> [w667 w670]
        frame False {
        }
        frame True {
        }
      }
      n177 = Bundle By Name(cluster=errorcluster {"status"=FALSE, "code"=0, "source"=""} ("error constant"), "status"=w663, "code"=w660, "source"=w658) -> (w656:errorcluster)
    }
  }
  "Error Out" <- w4
  "All_ERD_Data_Bundled_Brass" <- w3
